vi "Data Server copyright.vi"   [LabVIEW 2010]
panel:
  # "Data Server:\nTCP-Based Data Provider"
  # "©2002 Monroe Weber-Shirk\nall rights reserved\nmw24@cornell.edu\nDocumentation available at:\nhttp://ceeserver.cee.cornell.edu/mw24/Software/\nCivil and Environmental Engineering\nCornell University"
  # "This software may be modified as needed by the end user \nprovided this copyright dialog is included."
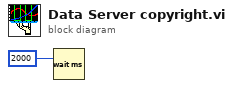
[diagram p0: block diagram]
diagram:
  n1 = Wait (ms)(milliseconds to wait=2000) -> ()  [unwired: 1 out]
